vi "BMU诊断标定.vi"(5 "timeout":u32, 6 "Socket":dbl, 7 "通用配置?":bool, 8 "CAN端口":u16(ring), 9 "设备索引号":u16(ring), 10 "CAN卡类型":u32(ring)=21, 11 "从板号":u8=1) -> (3 "成功?":bool)   [LabVIEW 2013] (continued)
                      n4644 = Transpose 2D Array(2D array=w6863) -> (transposed array=w6861:string[][])
                    }
                  }
                  n4645 = Insert Into Array(array=w6710, index (col)=2 ("禁用的索引 (列)"), new element #1=w6708, new element #2=w6707) -> (w6709:string[][])  [unwired: 1 in]
                }
              }
              n4646 = call "当前时间解析-8.6.vi"() -> ("名称格式时间"=w6501:string)  [unwired: 1 in, 18 out]
              n4647 = Concatenate Strings(w6501, w6500) -> (w6498:string)
              n4648 = call <vilib>:"Application Directory.vi"() -> ("Application Directory"=w6495:path)
              n4649 = call "文件对话框2"("start path"=w6495, "prompt"="选择保存的路径", "default name"=w6498) -> ("selected path"=w6496:path, "cancelled"=w6494:bool, "error out"=w6493:errorcluster)  [unwired: 9 in, 1 out]
              n4650 = call <vilib>:"Clear Errors.vi"("error in (no error)"=w6493) -> ()  [unwired: 6 in, 1 out]
              n4651 = case shown="假" w6494 {
                tunnel: w6502 -> [w6507 _]
                tunnel: w6496 -> [w6503 _]
                frame False {
                  n4652 = call-poly <vilib>:"Write To Spreadsheet File.vi"("append to file? (new file:F)"=FALSE, "2D data"=w6507, "file path (dialog if empty)"=w6503) -> ("new file path (Not A Path if cancelled)"=w6505:path)  [unwired: 3 in, 2 out]
                  n4653 = Path To String(path=w6505) -> (string=w6504:string)
                  n4654 = stacked-sequence {
                    tunnel: w6504 -> [w6510]
                    frame #0 {
                      n4655 = Concatenate Strings("保存完成,路径为:" ("字符串"), w6510) -> (w6511:string)
                      n4656 = One Button Dialog(message=w6511, button name ("OK")="是" ("按钮名称（“确定”）")) -> ()  [unwired: 1 out]
                    }
                  }
                }
                frame True {
                }
              }
            }
            frame Disabled {
              n4657 = stacked-sequence {
                seq-local: [w6881] -> [_]
                frame #0 {
                  n4658 = local read "项目信息"() -> (w6883:string[][])
                  n4659 = local read "项目信息2"() -> (w6880:T9)
                  n4660 = Array Subset(array=w6883, index (row)=0 ("索引"), index (col)=0 ("索引"), length (col)=2 ("索引")) -> (w6886:string[][])  [unwired: 1 in]
                  n4661 = local read "一级故障"() -> ()  [unwired: 1 out]
                  n4662 = local read "从板个数"() -> (w6881:dbl)
                  n4663 = Unbundle(w6880) -> ("电池额定容量(A)"=w6879:dbl, "电池实际容量(A)"=w6878:dbl, "车架(牌)号"=w6872:string, "配置文件版本"=w6871:string, "SOH(%)"=w6876:dbl, "SOC(%)"=w6877:dbl, "产品编号"=w6873:string)  [unwired: 2 out]
                  n4664 = Index Array(array=w6886, index (col) #1=1 ("禁用的索引 (列)"), index (col) #2=0 ("索引 (列)")) -> (element #1=w6870:string[], element #2=w6869:string[])  [unwired: 2 in]
                  n4665 = Build Array(w6879, w6878, w6877, w6876) -> (w6875:dbl[])
                  n4666 = Number To Decimal String(number=w6881) -> ()  [unwired: 1 in, 1 out]
                  n4667 = for {
                    tunnel: w6875 -> [w6891] mode=indexing
                    tunnel: [w6890] -> w6874 mode=indexing
                    n4668 = Format Into String(format string="%#f" ("格式字符串"), w6891) -> (resulting string=w6890:string)  [unwired: 2 in, 1 out]
                  }
                  n4669 = Insert Into Array(array=w6874, new element #1=w6873, new element #2=w6872, new element #3=w6871, new element #4=w6870) -> ()  [unwired: 1 in, 1 out]
                  n4670 = Insert Into Array(array=string[] ["电池额定容量", "电池实际容量", "SOC", "SOH", "产品编号", "车架(牌)号", "配置文件版本"], new element=w6869) -> ()  [unwired: 1 in, 1 out]
                }
              }
            }
          }
        }
        frame "读配置文件" {
        }
      }
    }
    frame Error {
    }
  }
  n4671 = while {
    tunnel: w73 -> [w6905]
    tunnel: w72 -> [w6904]
    tunnel: [w6903] -> w76
    tunnel: [w6902] -> w75
    tunnel: w41 -> [_]
    tunnel: w36 -> [w6895]
    stop <- w6892 stop-if-true
    n4672 = local read "timeout"() -> (w6893:bool)
    n4673 = local read "设备索引号"() -> (w6899:u16)
    n4674 = local read "CAN卡类型"() -> (w6900:u32)
    n4675 = local read "CAN端口"() -> (w6898:u16)
    n4676 = local read "停止"() -> (w6894:bool)
    n4677 = call "receiver-8.6.vi"("错误输入（无错误）"=w6895, "CAN端口"=w6898, "设备索引号"=w6899, "CAN卡类型"=w6900) -> ("错误输出"=w6901:errorcluster, "输出簇"=w6897:T30, "接收成功"=w6896:bool)  [unwired: 3 out]
    n4678 = Or(x=w6893, y=w6894) -> (x .or. y?=w6892:bool)
    n4679 = call <vilib>:"Clear Errors.vi"("error in (no error)"=w6901) -> ()  [unwired: 6 in, 1 out]
    n4680 = case shown="真" w6896 {
      tunnel: w6904 -> [w6906 w6912]
      tunnel: w6897 -> [_ w6911]
      tunnel: w6905 -> [w6907 w6910]
      tunnel: [w6907 w6909] -> w6903
      tunnel: [w6906 w6908] -> w6902
      frame False {
      }
      frame True {
        n4681 = Enqueue Element(queue=w6910, element=w6911, error in (no error)=w6912) -> (queue out=w6909:refnum<queue>, error out=w6908:errorcluster)  [unwired: 2 out]
      }
    }
  }
  n4682 = local write "面板选择"(T7."读写参数" ("面板选择")) -> ()
  n4683 = Release Queue(queue=w76, force destroy? (F)=TRUE ("强制销毁？(F)"), error in (no error)=w75) -> (error out=w78:errorcluster)  [unwired: 2 out]
  n4684 = call <vilib>:"Clear Errors.vi"("error in (no error)"=w78) -> ()  [unwired: 7 out]
